vi "Display Text from JSON.vi"(5 "No Error on Empty Input String":bool, 7 "Alphabetical Sort Objects":bool, 8 "error in (no error)":errorcluster, 10 "Offset":i32, 11 "Input JSON":string) -> (0 "error out":errorcluster, 1 "Offset after first JSON Value":i32, 3 "Display Text":string)   [LabVIEW 2019, in "JSONtext.lvlib"]
doc: "Reformate JSON as a more human-readable text string, for use in displays. The format is similar to YAML, but may not be fully compliant with that format."
uses:
  JSONtext.lvlib
  Parsing/Advance past Line Ending.vi
  String Subset.vi
  support/Unescape JSON string.vi
  <vilib>/Utility/error.llb/Error Cluster From Error Code.vi
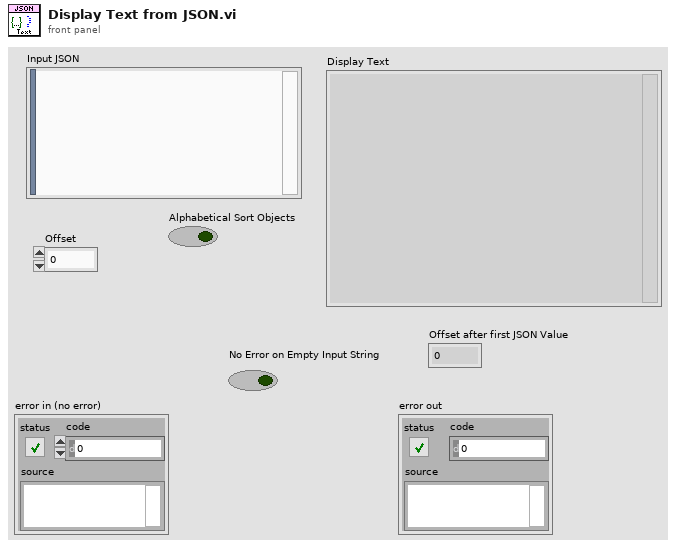
[diagram p1: front panel]
types:
  T1 = typedef "JSONtext.lvlib/Parsing State.ctl" = enum16{"Parser Error", "Object", "Array", "String", "Number/Other", "Leading Whitespace", "Object end", "Array end", "Value end"}
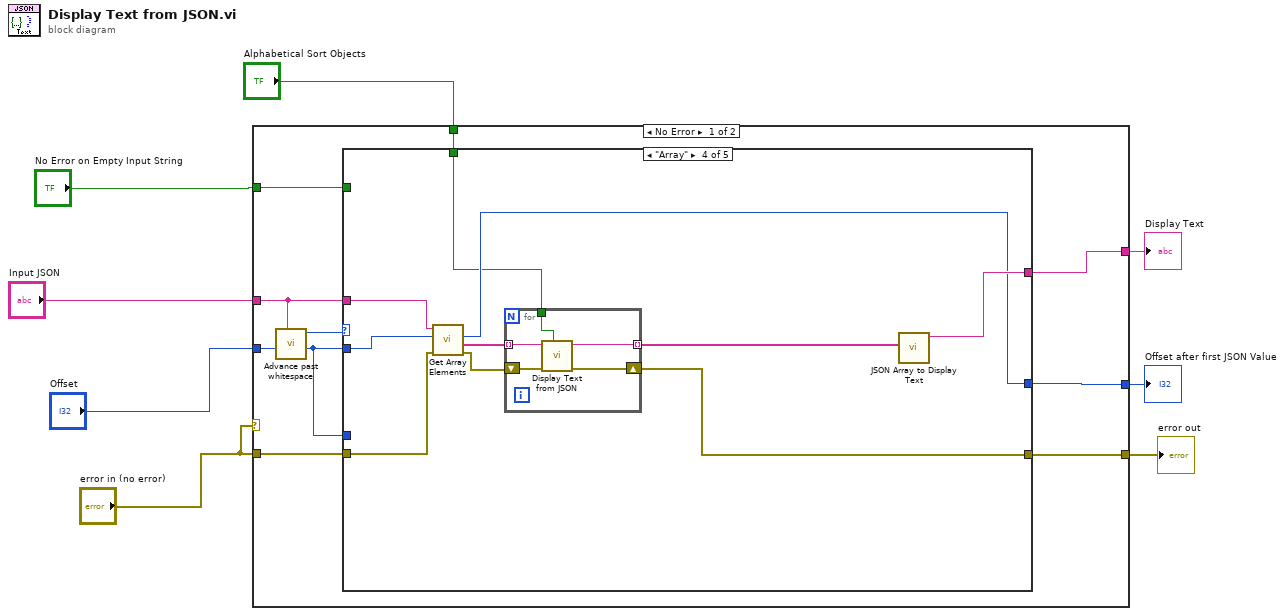
[diagram p0: block diagram]
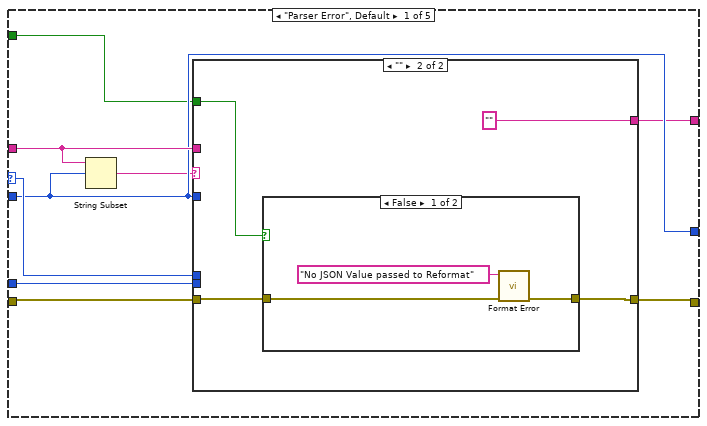
[diagram p2: hidden frame]
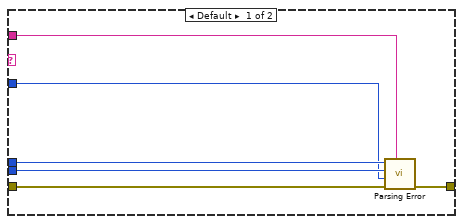
[diagram p3: hidden frame]
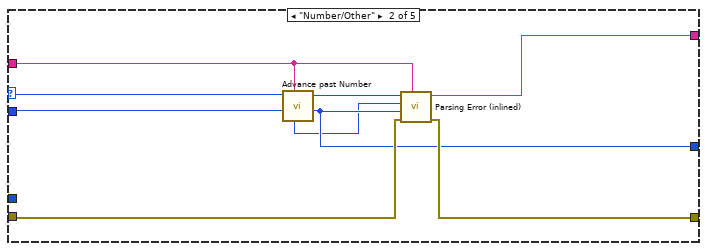
[diagram p5: hidden frame]
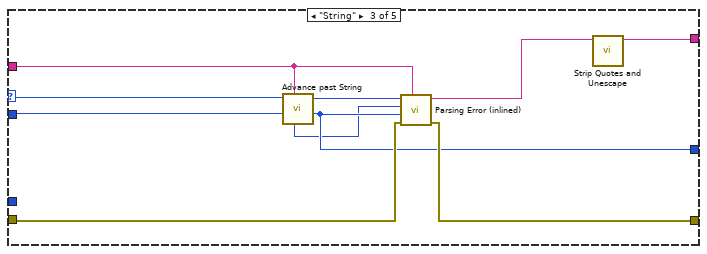
[diagram p6: hidden frame]
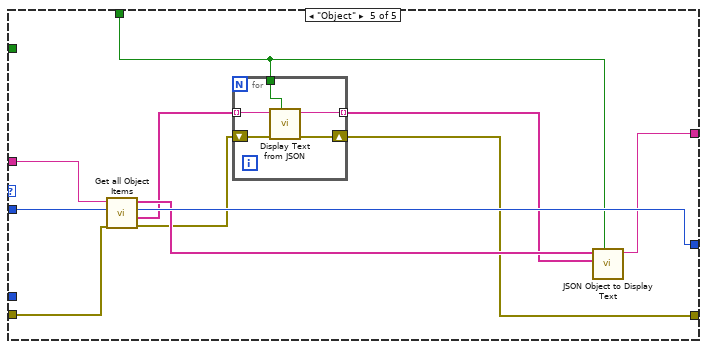
[diagram p7: hidden frame]
diagram:
  n1 = case shown="No Error" "error in (no error)" {
    tunnel: "Input JSON" -> [w18 _]
    tunnel: "Offset" -> [w16 w93]
    tunnel: [w15 w92] -> w6
    tunnel: "error in (no error)" -> [w14 w92]
    tunnel: [w12 _] -> w5
    tunnel: [w11 w93] -> w4
    tunnel: "Alphabetical Sort Objects" -> [w10 _]
    tunnel: "No Error on Empty Input String" -> [w9 _]
    frame No Error {
      n2 = call "Advance past whitespace.vi"("JSON"=w18, "Offset"=w16) -> ("Offset of first non-whitespace"=w13:i32, "Parser State"=w17:T1)  [unwired: 7 in, 1 out]
      n3 = case shown="\"Array\"" w17 {
        selector: w17 -> [w25 w50 w60 _ _]
        tunnel: w18 -> [w23 w43 w53 w70 w83]
        tunnel: w13 -> [w22 w49 w59 w69 w86]
        tunnel: [w22 w46 w56 w64 w85] -> w11
        tunnel: [w20 w42 w51 w67 w82] -> w12
        tunnel: [w27 w47 w57 w61 w76] -> w15
        tunnel: w14 -> [w26 w48 w58 w65 w78]
        tunnel: w13 -> [w24 _ _ _ _]
        tunnel: w10 -> [_ _ _ w62 w77]
        tunnel: w9 -> [w19 _ _ _ _]
        frame "Parser Error", Default {
          n4 = String Subset(string=w23, offset (0)=w22) -> (substring=w21:string)  [unwired: 1 in]
          n5 = case shown="\"\"" w21 {
            tunnel: [w33 w35] -> w27
            tunnel: w26 -> [w32 w36]
            tunnel: w25 -> [w31 _]
            tunnel: w24 -> [w30 _]
            tunnel: w23 -> [w29 _]
            tunnel: w22 -> [w28 _]
            tunnel: [_ ""] -> w20
            tunnel: w19 -> [_ w34]
            frame Default {
              n6 = call "Parsing Error.vi"("JSON"=w29, "error in (no error)"=w32, "Offset past match"=w28, "Value start"=w30, "State"=w31) -> ("error out"=w33:errorcluster)  [unwired: 6 in]
            }
            frame "" {
              n7 = case shown="False" w34 {
                tunnel: w36 -> [w40 w41]
                tunnel: [w39 w41] -> w35
                frame False {
                  n8 = call "Format Error.vi"("error in (no error)"=w40, "error message"="No JSON Value passed to Reformat") -> ("error out"=w39:errorcluster)  [unwired: 9 in]
                }
                frame True {
                }
              }
            }
          }
        }
        frame "Number/Other" {
          n9 = call "Advance past Number.vi"("JSON"=w43, "Offset (0)"=w49, "Parser State in"=w50) -> ("Offset past match"=w46:i32, "Parser State"=w44:T1, "Value start out"=w45:i32)  [unwired: 5 in, 1 out]
          n10 = call "Parsing Error (inlined).vi"("JSON"=w43, "error in (no error)"=w48, "Offset past match"=w46, "Value start"=w45, "State"=w44) -> ("error out"=w47:errorcluster, "Value (if no error)"=w42:string)  [unwired: 5 in]
        }
        frame "String" {
          n11 = call "Advance past String.vi"("JSON"=w53, "Offset"=w59, "State in"=w60) -> ("Offset past match"=w56:i32, "State"=w54:T1, "Value start out"=w55:i32)  [unwired: 6 in]
          n12 = call "Parsing Error (inlined).vi"("JSON"=w53, "error in (no error)"=w58, "Offset past match"=w56, "Value start"=w55, "State"=w54) -> ("error out"=w57:errorcluster, "Value (if no error)"=w52:string)  [unwired: 5 in]
          n13 = call "Strip Quotes and Unescape.vi"("String"=w52) -> ("result string"=w51:string)  [unwired: 9 in, 1 out]
        }
        frame "Array" {
          n14 = call "Get Array Elements.vi"("error in (no error)"=w65, "Offset"=w69, "JSON"=w70) -> ("error out"=w66:errorcluster, "<JSON>"=w68:string[], "Offset past"=w64:i32)  [unwired: 6 in]
          n15 = for {
            tunnel: w68 -> [w75] mode=indexing
            tunnel: [w74] -> w63 mode=indexing
            shift-right: [w72] -> w61
            shift-left: w66 -> [w73]
            tunnel: w62 -> [w71]
            n16 = call "Display Text from JSON.vi"("Alphabetical Sort Objects"=w71, "error in (no error)"=w73, "Input JSON"=w75) -> ("error out"=w72:errorcluster, "Display Text"=w74:string)  [unwired: 6 in, 1 out]
          }
          n17 = call "JSON Array to Display Text.vi"("Array of JSON Text"=w63) -> ("Display Text"=w67:string)  [unwired: 10 in]
        }
        frame "Object" {
          n18 = call "Get all Object Items.vi"("error in (no error)"=w78, "Offset"=w86, "JSON"=w83) -> ("error out"=w79:errorcluster, "<JSON>"=w81:string[], "Offset past"=w85:i32, "Item Names"=w84:string[])  [unwired: 5 in]
          n19 = for {
            tunnel: w81 -> [w91] mode=indexing
            tunnel: [w90] -> w80 mode=indexing
            shift-right: [w88] -> w76
            shift-left: w79 -> [w89]
            tunnel: w77 -> [w87]
            n20 = call "Display Text from JSON.vi"("Alphabetical Sort Objects"=w87, "error in (no error)"=w89, "Input JSON"=w91) -> ("error out"=w88:errorcluster, "Display Text"=w90:string)  [unwired: 6 in, 1 out]
          }
          n21 = call "JSON Object to Display Text.vi"("Alphabetical Sort"=w77, "elements"=w80, "Names"=w84) -> ("Display Text"=w82:string)  [unwired: 8 in]
        }
      }
    }
    frame Error {
    }
  }
  "Offset after first JSON Value" <- w4
  "Display Text" <- w5
  "error out" <- w6
